vi "Start Processes.vi"(8 "error in (no error)":errorcluster, 11 "Execution UI In":refnum<class "Execution UI.lvclass">) -> (0 "error out":errorcluster, 3 "Execution UI Out":refnum<class "Execution UI.lvclass">)   [LabVIEW 2020, in "Execution UI.lvclass"]
uses:
  Execution UI.lvclass
  Test Runner/Test Runner.lvclass
  Report Generator/Report Generator.lvclass
  Application Framework/Process Classes/Process/Process.lvclass
  Icon Decorator/Icon Decorator.lvclass
  C:/Git/astemes-lunit/source/Application Framework/Process Classes/Process/Process.lvclass
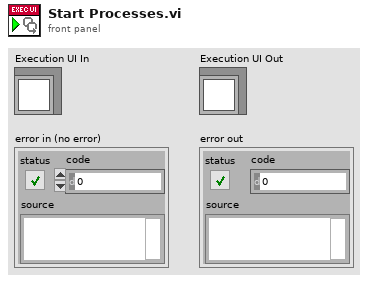
[diagram p1: front panel]
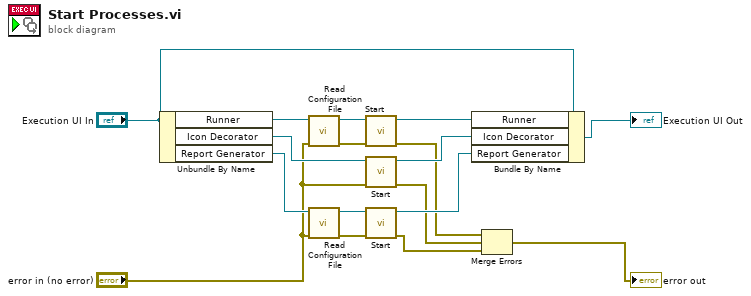
[diagram p0: block diagram]
diagram:
  n1 = Unbundle By Name("Execution UI In") -> ("Runner"=w15:refnum<class "Test Runner.lvclass">, "Icon Decorator"=w12:refnum<class "Icon Decorator.lvclass">, "Report Generator"=w11:refnum<class "Report Generator.lvclass">)
  n2 = call "Read Configuration File.vi"("error in (no error)"="error in (no error)", "Test Runner in"=w15) -> ("error out"=w8:errorcluster, "Test Runner out"=w14:refnum<class "Test Runner.lvclass">)  [unwired: 8 in]
  n3 = call "Read Configuration File.vi"("error in (no error)"="error in (no error)", "Report Generator In"=w11) -> ("error out"=w7:errorcluster, "Report Generator Out"=w13:refnum<class "Report Generator.lvclass">)  [unwired: 8 in]
  n4 = call "Start.vi"("error in (no error)"=w8, "Process In"=w14) -> ("error out"=w5:errorcluster, "Process Out"=w17:refnum<class "Test Runner.lvclass">)  [unwired: 8 in]
  n5 = call "Start.vi"("error in (no error)"="error in (no error)", "Process In"=w12) -> ("error out"=w4:errorcluster, "Process Out"=w10:refnum<class "Icon Decorator.lvclass">)  [unwired: 8 in]
  n6 = call "Start.vi"("error in (no error)"=w7, "Process In"=w13) -> ("error out"=w3:errorcluster, "Process Out"=w9:refnum<class "Report Generator.lvclass">)  [unwired: 8 in]
  n7 = Bundle By Name(cluster="Execution UI In", "Runner"=w17, "Icon Decorator"=w10, "Report Generator"=w9) -> (→"Execution UI Out":refnum<class "Execution UI.lvclass">)
  n8 = Merge Errors(w5, w4, w3) -> (→"error out":errorcluster)
